vi "Send Load Pattern.vi"(7 "Message Priority (Normal)":T2=enum."Normal", 8 "error in (no error)":errorcluster, 10 "PatternData":T1(array[cluster]), 11 "Message Enqueuer":refnum<class "Message Enqueuer.lvclass">) -> (0 "error out":errorcluster, 3 "Message Enqueuer out":refnum<class "Message Enqueuer.lvclass">)   [LabVIEW 2015, in "CS++PPG.lvlib" / "Load Pattern Msg.lvclass"]
doc: "Sends the <B>CS++PPG.lvlib:Load Pattern Msg.lvclass</B> message.\n\n<B>CS++PPG.lvlib:CS++PPG.lvclass:Load Pattern.vi</B> Description:\n\nThis VI loads a pattern to the pulsed pattern generator. Afterwards the PPG device should be ready to start."
uses:
  Load Pattern Msg.lvclass
  <vilib>/ActorFramework/Message Enqueuer/Message Enqueuer.lvclass
  <vilib>/ActorFramework/Message Enqueuer/Message Priority.ctl
  Load Pattern Msg.lvclass/Load Pattern Msg.ctl
  <vilib>/ActorFramework/Message Enqueuer/Message Enqueuer.lvclass/Message Enqueuer.ctl
  <vilib>/ActorFramework/Message Priority Queue/Priority Enqueue.vi
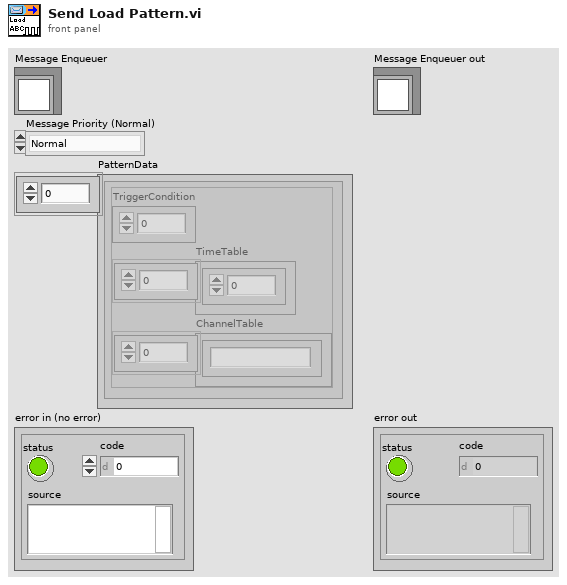
[diagram p1: front panel]
types:
  T1 = cluster{"TriggerCondition":i32, "TimeTable":dbl[], "ChannelTable":string[]}[]
  T2 = typedef "Actor Framework.lvlib/Message Enqueuer.lvclass/Message Priority.ctl" = enum16{"Low", "Normal", "High"}
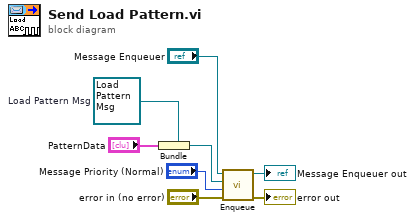
[diagram p0: block diagram]
diagram:
  w2 = refnum<class "Load Pattern Msg.lvclass"> refnum  # Load Pattern Msg
  n1 = Bundle(cluster=w2, "PatternData") -> (w5:refnum<class "Load Pattern Msg.lvclass">)
  n2 = call <vilib>:"Enqueue.vi"("error in (no error)"="error in (no error)", "Message Priority (Normal)"="Message Priority (Normal)", "Message"=w5, "Message Enqueuer in"="Message Enqueuer") -> ("error out"=→"error out":errorcluster, "Message Enqueuer out"=→"Message Enqueuer out":refnum<class "Message Enqueuer.lvclass">)  [unwired: 6 in]
